vi "ql2proto_query_type_compose.vi"(9 "global options (key,val)":string[][](array[string]), 10 "query":string, 11 "query_type":T1) -> (3 "tcp_write":string)   [LabVIEW 2017]
uses:
  ql2proto_query_type.ctl
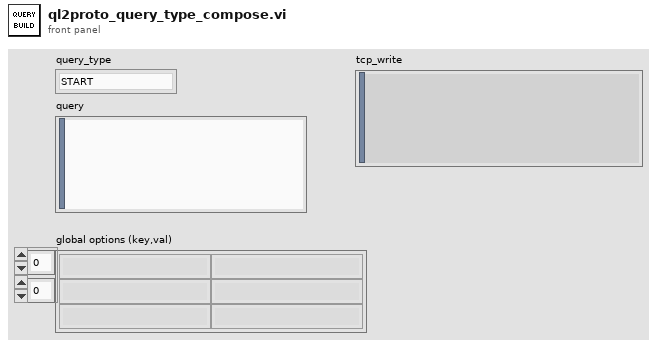
[diagram p1: front panel]
types:
  T1 = typedef "ql2proto_query_type.ctl" = enum8{"START", "CONTINUE", "STOP", "NOREPLY_WAIT", "SERVER_INFO", "invalid"}
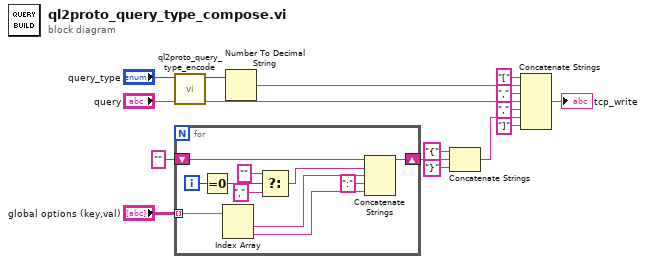
[diagram p0: block diagram]
diagram:
  n1 = call "ql2proto_query_type_encode.vi"("query_type"="query_type") -> ("id"=w14:u32)  [unwired: 9 in, 1 out]
  n2 = for {
    tunnel: "global options (key,val)" -> [w19] mode=indexing
    shift-right: [w21] -> w8
    shift-left: "" -> [w26]
    i -> [w25]
    n3 = Equal To 0?(x=w25) -> (x = 0?=w24:bool)
    n4 = Index Array(array=w19) -> (element #1=w18:string, element #2=w16:string)  [unwired: 2 in]
    n5 = Select(t="", s=w24, f=",") -> (s? t:f=w20:string)
    n6 = Concatenate Strings(w26, w20, w18, ":" ("string"), w16) -> (w21:string)
  }
  n7 = Number To Decimal String(number=w14) -> (decimal integer string=w13:string)  [unwired: 1 in]
  n8 = Concatenate Strings("{" ("string"), w8, "}" ("string")) -> (w5:string)
  n9 = Concatenate Strings("[" ("string"), w13, "," ("string"), "query", "," ("string"), w5, "]" ("string")) -> (→"tcp_write":string)
